vi "test_read-nmea-data2.vi"() -> ()   [LabVIEW 2019] (continued)
\tF9P\t\t\n15:11:49.05\tF9P\t\t\n15:11:49.07\tF9P\t\t\n15:11:49.09\tF9P\t\t\n15:11:49.11\tF9P\t\t\n15:11:49.13\tF9P\t\t\n15:11:49.15\tF9P\t\t\n15:11:49.17\tF9P\t\t\n15:11:49.19\tF9P\t\t\n15:11:49.21\tF9P\t\t\n15:11:49.23\tF9P\t\t\n15:11:49.25\tF9P\t$GNRMC,061151.00,A,3723.52582,N,12656.91812,E,3.101,50.80,250720,,,A,V*3C\n\t\n15:11:49.27\tF9P\t$GNVTG,50.80,T,,M,3.101,N,5.743,K,A*18\n\t\n15:11:49.29\tF9P\t$GNGGA,061151.00,3723.52582,N,12656.91812,E,1,12,0.68,36.2,M,18.5,M,,*7E\n\t\n15:11:49.31\tF9P\t$GNGSA,A,3,12,06,19,05,17,09,04,02,,,,,1.27,0.68,1.08,1*03\n\t\n15:11:49.33\tF9P\t$GNGSA,A,3,85,71,84,,,,,,,,,,1.27,0.68,1.08,2*06\n\t\n15:11:49.35\tF9P\t$GNGSA,A,3,36,19,11,04,09,12,,,,,,,1.27,0.68,1.08,3*03\n\t\n15:11:49.37\tF9P\t$GNGSA,A,3,14,11,33,,,,,,,,,,1.27,0.68,1.08,4*02\n\t\n15:11:49.39\tF9P\t$GPGSV,3,1,09,02,54,318,38,04,18,044,21,05,37,247,31,06,64,047,31,1*64\n\t\n15:11:49.41\tF9P\t$GPGSV,3,2,09,09,45,074,30,12,24,277,31,17,33,153,31,19,53,157,32,1*6E\n\t\n15:11:49.43\tF9P\t$GPGSV,3,3,09,25,12,307,16,1*5A\n\t\n15:11:49.45\tF9P\t$GPGSV,3,1,09,02,54,318,,04,18,044,13,05,37,247,16,06,64,047,28,6*64\n\t\n15:11:49.47\tF9P\t$GPGSV,3,2,09,09,45,074,30,12,24,277,21,17,33,153,23,19,53,157,,6*6A\n\t\n15:11:49.49\tF9P\t$GPGSV,3,3,09,25,12,307,,6*5A\n\t\n15:11:49.51\tF9P\t$GLGSV,2,1,08,69,12,031,,70,71,039,,71,52,205,44,72,04,209,,1*7A\n\t\n15:11:49.53\tF9P\t$GLGSV,2,2,08,77,01,326,,84,20,122,11,85,70,067,38,86,37,330,,1*73\n\t\n15:11:49.55\tF9P\t$GLGSV,2,1,08,69,12,031,,70,71,039,,71,52,205,21,72,04,209,,3*7B\n\t\n15:11:49.57\tF9P\t$GLGSV,2,2,08,77,01,326,,84,20,122,15,85,70,067,22,86,37,330,,3*7E\n\t\n15:11:49.59\tF9P\t$GAGSV,2,1,08,02,08,297,10,04,66,118,28,09,32,193,34,11,71,358,26,7*71\n\t\n15:11:49.61\tF9P\t$GAGSV,2,2,08,12,40,102,27,19,26,045,32,25,09,249,,36,26,308,32,7*7C\n\t\n15:11:49.63\tF9P\t$GAGSV,2,1,08,02,08,297,,04,66,118,,09,32,193,32,11,71,358,,2*7D\n\t\n15:11:49.65\tF9P\t$GAGSV,2,2,08,12,40,102,,19,26,045,,25,09,249,,36,26,308,,2*7C\n\t\n15:11:49.67\tF9P\t$GBGSV,1,1,03,11,50,132,31,14,87,127,28,33,60,219,34,1*4D\n\t\n15:11:49.69\tF9P\t$GBGSV,1,1,03,11,50,132,28,14,87,127,35,33,60,219,,3*4C\n\t\n15:11:49.71\tF9P\t$GNGLL,3723.52582,N,12656.91812,E,061151.00,A,A*7D\n\t\n15:11:49.73\tF9P\t\t\n15:11:49.75\tF9P\t\t\n15:11:49.77\tF9P\t\t\n15:11:49.79\tF9P\t\t\n15:11:49.81\tF9P\t\t\n15:11:49.83\tF9P\t\t\n15:11:49.85\tF9P\t\t\n15:11:49.87\tF9P\t\t\n15:11:49.89\tF9P\t\t\n15:11:49.91\tF9P\t\t\n15:11:49.93\tF9P\t\t\n15:11:49.95\tF9P\t\t\n15:11:49.97\tF9P\t\t\n15:11:49.99\tF9P\t\t\n15:11:50.01\tF9P\t\t\n15:11:50.03\tF9P\t\t\n15:11:50.05\tF9P\t\t\n15:11:50.07\tF9P\t\t\n15:11:50.09\tF9P\t\t\n15:11:50.11\tF9P\t\t\n15:11:50.13\tF9P\t\t\n15:11:50.15\tF9P\t\t\n15:11:50.17\tF9P\t\t\n15:11:50.19\tF9P\t\t\n15:11:50.21\tF9P\t\t\n15:11:50.23\tF9P\t\t\n15:11:50.25\tF9P\t$GNRMC,061152.00,A,3723.52625,N,12656.91894,E,2.824,51.00,250720,,,A,V*39\n\t\n15:11:50.27\tF9P\t$GNVTG,51.00,T,,M,2.824,N,5.229,K,A*17\n\t\n15:11:50.29\tF9P\t$GNGGA,061152.00,3723.52625,N,12656.91894,E,1,12,0.68,35.8,M,18.5,M,,*74\n\t\n15:11:50.31\tF9P\t$GNGSA,A,3,12,06,19,05,17,09,04,02,,,,,1.27,0.68,1.08,1*03\n\t\n15:11:50.33\tF9P\t$GNGSA,A,3,85,71,84,,,,,,,,,,1.27,0.68,1.08,2*06\n\t\n15:11:50.35\tF9P\t$GNGSA,A,3,36,19,11,04,09,12,,,,,,,1.27,0.68,1.08,3*03\n\t\n15:11:50.37\tF9P\t$GNGSA,A,3,14,11,33,,,,,,,,,,1.27,0.68,1.08,4*02\n\t\n15:11:50.39\tF9P\t$GPGSV,3,1,09,02,54,318,39,04,18,044,,05,37,247,26,06,64,047,32,1*63\n\t\n15:11:50.41\tF9P\t$GPGSV,3,2,09,09,45,074,30,12,24,277,28,17,33,153,30,19,53,157,34,1*61\n\t\n15:11:50.43\tF9P\t$GPGSV,3,3,09,25,12,307,17,1*5B\n\t\n15:11:50.45\tF9P\t$GPGSV,3,1,09,02,54,318,,04,18,044,14,05,37,247,17,06,64,047,29,6*63\n\t\n15:11:50.47\tF9P\t$GPGSV,3,2,09,09,45,074,32,12,24,277,20,17,33,153,24,19,53,157,,6*6E\n\t\n15:11:50.49\tF9P\t$GPGSV,3,3,09,25,12,307,,6*5A\n\t\n15:11:50.51\tF9P\t$GLGSV,2,1,08,69,12,031,,70,71,039,,71,52,205,48,72,04,209,,1*76\n\t\n15:11:50.53\tF9P\t$GLGSV,2,2,08,77,01,326,,84,20,122,12,85,70,067,35,86,37,330,,1*7D\n\t\n15:11:50.55\tF9P\t$GLGSV,2,1,08,69,12,031,,70,71,039,,71,52,205,22,72,04,209,,3*78\n\t\n15:11:50.57\tF9P\t$GLGSV,2,2,08,77,01,326,,84,20,122,15,85,70,067,21,86,37,330,,3*7D\n\t\n15:11:50.59\tF9P\t$GAGSV,2,1,08,02,08,297,08,04,66,118,29,09,32,193,34,11,71,358,26,7*79\n\t\n15:11:50.61\tF9P\t$GAGSV,2,2,08,12,40,102,26,19,26,045,31,25,09,249,,36,26,308,23,7*7E\n\t\n15:11:50.63\tF9P\t$GAGSV,2,1,08,02,08,297,,04,66,118,,09,32,193,33,11,71,358,,2*7C\n\t\n15:11:50.65\tF9P\t$GAGSV,2,2,08,12,40,102,,19,26,045,,25,09,249,,36,26,308,,2*7C\n\t\n15:11:50.67\tF9P\t$GBGSV,1,1,03,11,50,132,30,14,87,127,32,33,60,219,37,1*44\n\t\n15:11:50.69\tF9P\t$GBGSV,1,1,03,11,50,132,,14,87,127,,33,60,219,,3*40\n\t\n15:11:50.71\tF9P\t$GNGLL,3723.52625,N,12656.91894,E,061152.00,A,A*7E\n\t\n15:11:50.73\tF9P\t\t\n15:11:50.75\tF9P\t\t\n15:11:50.77\tF9P\t\t\n15:11:50.79\tF9P\t\t\n15:11:50.81\tF9P\t\t\n15:11:50.83\tF9P\t\t\n15:11:50.85\tF9P\t\t\n15:11:50.87\tF9P\t\t\n15:11:50.89\tF9P\t\t\n15:11:50.91\tF9P\t\t\n15:11:50.93\tF9P\t\t\n15:11:50.95\tF9P\t\t\n15:11:50.97\tF9P\t\t\n15:11:50.99\tF9P\t\t\n15:11:51.01\tF9P\t\t\n15:11:51.03\tF9P\t\t\n15:11:51.05\tF9P\t\t\n15:11:51.07\tF9P\t\t\n15:11:51.09\tF9P\t\t\n15:11:51.11\tF9P\t\t\n15:11:51.13\tF9P\t\t\n15:11:51.15\tF9P\t\t\n15:11:51.17\tF9P\t\t\n15:11:51.19\tF9P\t\t\n15:11:51.21\tF9P\t\t\n15:11:51.23\tF9P\t\t\n15:11:51.25\tF9P\t$GNRMC,061153.00,A,3723.52665,N,12656.91962,E,2.290,47.20,250720,,,A,V*34\n\t\n15:11:51.27\tF9P\t$GNVTG,47.20,T,,M,2.290,N,4.241,K,A*18\n\t\n15:11:51.29\tF9P\t$GNGGA,061153.00,3723.52665,N,12656.91962,E,1,12,0.71,35.0,M,18.5,M,,*79\n\t\n15:11:51.31\tF9P\t$GNGSA,A,3,12,06,19,05,17,09,04,02,,,,,1.31,0.71,1.10,1*05\n\t\n15:11:51.33\tF9P\t$GNGSA,A,3,85,71,84,,,,,,,,,,1.31,0.71,1.10,2*00\n\t\n15:11:51.35\tF9P\t$GNGSA,A,3,36,19,11,04,09,12,,,,,,,1.31,0.71,1.10,3*05\n\t\n15:11:51.37\tF9P\t$GNGSA,A,3,14,11,33,,,,,,,,,,1.31,0.71,1.10,4*04\n\t\n15:11:51.39\tF9P\t$GPGSV,3,1,09,02,54,318,41,04,18,044,23,05,37,247,26,06,64,047,32,1*6D\n\t\n15:11:51.41\tF9P\t$GPGSV,3,2,09,09,45,074,34,12,24,277,28,17,33,153,34,19,53,157,33,1*66\n\t\n15:11:51.43\tF9P\t$GPGSV,3,3,09,25,12,307,16,1*5A\n\t\n15:11:51.45\tF9P\t$GPGSV,3,1,09,02,54,318,,04,18,044,15,05,37,247,16,06,64,047,32,6*69\n\t\n15:11:51.47\tF9P\t$GPGSV,3,2,09,09,45,074,26,12,24,277,18,17,33,153,23,19,53,157,,6*67\n\t\n15:11:51.49\tF9P\t$GPGSV,3,3,09,25,12,307,,6*5A\n\t\n15:11:51.51\tF9P\t$GLGSV,2,1,08,69,12,031,,70,71,039,,71,52,205,41,72,04,209,,1*7F\n\t\n15:11:51.53\tF9P\t$GLGSV,2,2,08,77,01,326,,84,20,122,11,85,70,067,31,86,37,330,,1*7A\n\t\n15:11:51.55\tF9P\t$GLGSV,2,1,08,69,12,031,,70,71,039,,71,52,205,24,72,04,209,,3*7E\n\t\n15:11:51.57\tF9P\t$GLGSV,2,2,08,77,01,326,,84,20,122,15,85,70,067,29,86,37,330,,3*75\n\t\n15:11:51.59\tF9P\t$GAGSV,2,1,08,02,08,297,12,04,66,118,29,09,32,193,37,11,71,358,31,7*77\n\t\n15:11:51.61\tF9P\t$GAGSV,2,2,08,12,40,102,32,19,26,045,24,25,09,249,,36,26,308,30,7*7D\n\t\n15:11:51.63\tF9P\t$GAGSV,2,1,08,02,08,297,,04,66,118,,09,32,193,,11,71,358,,2*7C\n\t\n15:11:51.65\tF9P\t$GAGSV,2,2,08,12,40,102,,19,26,045,,25,09,249,,36,26,308,,2*7C\n\t\n15:11:51.67\tF9P\t$GBGSV,1,1,03,11,50,132,24,14,87,127,33,33,60,219,38,1*4F\n\t\n15:11:51.69\tF9P\t$GBGSV,1,1,04,08,,,32,11,50,132,,14,87,127,,33,60,219,,3*4E\n\t\n15:11:51.71\tF9P\t$GNGLL,3723.52665,N,12656.91962,E,061153.00,A,A*73\n\t\n15:11:51.73\tF9P\t\t\n15:11:51.75\tF9P\t\t\n15:11:51.77\tF9P\t\t\n15:11:51.79\tF9P\t\t\n15:11:51.81\tF9P\t\t\n15:11:51.83\tF9P\t\t\n15:11:51.85\tF9P\t\t\n15:11:51.87\tF9P\t\t\n15:11:51.89\tF9P\t\t\n15:11:51.91\tF9P\t\t\n15:11:51.93\tF9P\t\t\n15:11:51.95\tF9P\t\t\n15:11:51.97\tF9P\t\t\n15:11:51.99\tF9P\t\t\n15:11:52.01\tF9P\t\t\n15:11:52.03\tF9P\t\t\n15:11:52.05\tF9P\t\t\n15:11:52.07\tF9P\t\t\n15:11:52.09\tF9P\t\t\n15:11:52.11\tF9P\t\t\n15:11:52.13\tF9P\t\t\n15:11:52.15\tF9P\t\t\n15:11:52.17\tF9P\t\t\n15:11:52.19\tF9P\t\t\n15:11:52.21\tF9P\t\t\n15:11:52.23\tF9P\t\t\n15:11:52.25\tF9P\t$GNRMC,061154.00,A,3723.52702,N,12656.92007,E,2.069,41.23,250720,,,A,V*3B\n\t\n15:11:52.27\tF9P\t$GNVTG,41.23,T,,M,2.069,N,3.832,K,A*10\n\t\n15:11:52.29\tF9P\t$GNGGA,061154.00,3723.52702,N,12656.92007,E,1,12,0.68,35.3,M,18.5,M,,*7C\n\t\n15:11:52.31\tF9P\t$GNGSA,A,3,12,06,19,05,17,09,04,02,,,,,1.27,0.68,1.08,1*03\n\t\n15:11:52.33\tF9P\t$GNGSA,A,3,85,71,84,,,,,,,,,,1.27,0.68,1.08,2*06\n\t\n15:11:52.35\tF9P\t$GNGSA,A,3,36,19,11,04,09,12,,,,,,,1.27,0.68,1.08,3*03\n\t\n15:11:52.37\tF9P\t$GNGSA,A,3,14,11,33,,,,,,,,,,1.27,0.68,1.08,4*02\n\t\n15:11:52.39\tF9P\t$GPGSV,3,1,09,02,55,319,43,04,18,044,22,05,37,247,27,06,64,047,33,1*6E\n\t\n15:11:52.41\tF9P\t$GPGSV,3,2,09,09,45,074,33,12,24,277,27,17,33,153,36,19,53,157,36,1*69\n\t\n15:11:52.43\tF9P\t$GPGSV,3,3,09,25,12,307,18,1*54\n\t\n15:11:52.45\tF9P\t$GPGSV,3,1,09,02,55,319,,04,18,044,17,05,37,247,15,06,64,047,27,6*6C\n\t\n15:11:52.47\tF9P\t$GPGSV,3,2,09,09,45,074,28,12,24,277,17,17,33,153,23,19,53,157,,6*66\n\t\n15:11:52.49\tF9P\t$GPGSV,3,3,09,25,12,307,,6*5A\n\t\n15:11:52.51\tF9P\t$GLGSV,2,1,08,69,12,031,,70,71,039,,71,52,205,44,72,04,209,,1*7A\n\t\n15:11:52.53\tF9P\t$GLGSV,2,2,08,77,01,326,,84,20,122,12,85,70,067,35,86,37,330,,1*7D\n\t\n15:11:52.55\tF9P\t$GLGSV,2,1,08,69,12,031,,70,71,039,,71,52,205,30,72,04,209,,3*7B\n\t\n15:11:52.57\tF9P\t$GLGSV,2,2,08,77,01,326,,84,20,122,15,85,70,067,28,86,37,330,,3*74\n\t\n15:11:52.59\tF9P\t$GAGSV,2,1,08,02,08,297,08,04,66,118,28,09,32,193,43,11,71,358,26,7*78\n\t\n15:11:52.61\tF9P\t$GAGSV,2,2,08,12,40,102,26,19,26,045,24,25,09,249,,36,26,308,29,7*70\n\t\n15:11:52.63\tF9P\t$GAGSV,2,1,08,02,08,297,,04,66,118,,09,32,193,,11,71,358,,2*7C\n\t\n15:11:52.65\tF9P\t$GAGSV,2,2,08,12,40,102,,19,26,045,,25,09,249,,36,26,308,,2*7C\n\t\n15:11:52.67\tF9P\t$GBGSV,1,1,03,11,50,132,29,14,87,127,31,33,60,219,40,1*4F\n\t\n15:11:52.69\tF9P\t$GBGSV,1,1,04,08,,,27,11,50,132,,14,87,127,,33,60,219,,3*4A\n\t\n15:11:52.71\tF9P\t$GNGLL,3723.52702,N,12656.92007,E,061154.00,A,A*7D\n\t\n15:11:52.73\tF9P\t\t\n15:11:52.75\tF9P\t\t\n15:11:52.77\tF9P\t\t\n15:11:52.79\tF9P\t\t\n15:11:52.81\tF9P\t\t\n15:11:52.83\tF9P\t\t\n15:11:52.85\tF9P\t\t\n15:11:52.87\tF9P\t\t\n15:11:52.89\tF9P\t\t\n15:11:52.91\tF9P\t\t\n15:11:52.93\tF9P\t\t\n15:11:52.95\tF9P\t\t\n15:11:52.97\tF9P\t\t\n15:11:52.99\tF9P\t\t\n15:11:53.01\tF9P\t\t\n15:11:53.03\tF9P\t\t\n15:11:53.05\tF9P\t\t\n15:11:53.07\tF9P\t\t\n15:11:53.09\tF9P\t\t\n15:11:53.11\tF9P\t\t\n15:11:53.13\tF9P\t\t\n15:11:53.15\tF9P\t\t\n15:11:53.17\tF9P\t\t\n15:11:53.19\tF9P\t\t\n15:11:53.21\tF9P\t\t\n15:11:53.23\tF9P\t\t\n15:11:53.25\tF9P\t$GNRMC,061155.00,A,3723.52737,N,12656.92072,E,2.566,49.21,250720,,,A,V*3E\n\t\n15:11:53.27\tF9P\t$GNVTG,49.21,T,,M,2.566,N,4.751,K,A*1D\n\t\n15:11:53.29\tF9P\t$GNGGA,061155.00,3723.52737,N,12656.92072,E,1,12,0.70,34.5,M,18.5,M,,*77\n\t\n15:11:53.31\tF9P\t$GNGSA,A,3,12,06,19,05,17,09,04,02,,,,,1.39,0.70,1.20,1*0F\n\t\n15:11:53.33\tF9P\t$GNGSA,A,3,85,70,71,84,,,,,,,,,1.39,0.70,1.20,2*0D\n\t\n15:11:53.35\tF9P\t$GNGSA,A,3,36,19,11,04,09,12,,,,,,,1.39,0.70,1.20,3*0F\n\t\n15:11:53.37\tF9P\t$GNGSA,A,3,14,11,33,,,,,,,,,,1.39,0.70,1.20,4*0E\n\t\n15:11:53.39\tF9P\t$GPGSV,3,1,09,02,55,319,39,04,18,044,25,05,37,247,26,06,64,047,34,1*62\n\t\n15:11:53.41\tF9P\t$GPGSV,3,2,09,09,45,074,33,12,24,277,26,17,33,153,40,19,53,157,33,1*6C\n\t\n15:11:53.43\tF9P\t$GPGSV,3,3,09,25,12,307,17,1*5B\n\t\n15:11:53.45\tF9P\t$GPGSV,3,1,09,02,55,319,,04,18,044,15,05,37,247,14,06,64,047,26,6*6E\n\t\n15:11:53.47\tF9P\t$GPGSV,3,2,09,09,45,074,33,12,24,277,14,17,33,153,24,19,53,157,,6*68\n\t\n15:11:53.49\tF9P\t$GPGSV,3,3,09,25,12,307,,6*5A\n\t\n15:11:53.51\tF9P\t$GLGSV,2,1,08,69,12,031,,70,71,039,32,71,52,205,45,72,04,209,,1*7A\n\t\n15:11:53.53\tF9P\t$GLGSV,2,2,08,77,01,326,,84,20,122,11,85,70,067,29,86,37,330,,1*73\n\t\n15:11:53.55\tF9P\t$GLGSV,2,1,08,69,12,031,,70,71,039,,71,52,205,30,72,04,209,,3*7B\n\t\n15:11:53.57\tF9P\t$GLGSV,2,2,08,77,01,326,,84,20,122,17,85,70,067,26,86,37,330,,3*78\n\t\n15:11:53.59\tF9P\t$GAGSV,2,1,08,02,08,297,12,04,66,118,29,09,32,193,33,11,71,358,26,7*75\n\t\n15:11:53.61\tF9P\t$GAGSV,2,2,08,12,40,102,27,19,26,045,25,25,09,249,,36,26,308,33,7*7B\n\t\n15:11:53.63\tF9P\t$GAGSV,2,1,08,02,08,297,,04,66,118,,09,32,193,,11,71,358,,2*7C\n\t\n15:11:53.65\tF9P\t$GAGSV,2,2,08,12,40,102,,19,26,045,,25,09,249,,36,26,308,,2*7C\n\t\n15:11:53.67\tF9P\t$GBGSV,1,1,03,11,50,132,29,14,87,127,26,33,60,219,33,1*4D\n\t\n15:11:53.69\tF9P\t$GBGSV,1,1,04,08,,,25,11,50,132,,14,87,127,,33,60,219,,3*48\n\t\n15:11:53.71\tF9P\t$GNGLL,3723.52737,N,12656.92072,E,061155.00,A,A*78\n\t\n15:11:53.73\tF9P\t\t\n15:11:53.75\tF9P\t\t\n15:11:53.77\tF9P\t\t\n15:11:53.79\tF9P\t\t\n15:11:53.81\tF9P\t\t\n15:11:53.83\tF9P\t\t\n15:11:53.85\tF9P\t\t\n15:11:53.87\tF9P\t\t\n15:11:53.89\tF9P\t\t\n15:11:53.91\tF9P\t\t\n15:11:53.93\tF9P\t\t\n15:11:53.95\tF9P\t\t\n15:11:53.97\tF9P\t\t\n15:11:53.99\tF9P\t\t\n15:11:54.01\tF9P\t\t\n15:11:54.03\tF9P\t\t\n15:11:54.05\tF9P\t\t\n15:11:54.07\tF9P\t\t\n15:11:54.09\tF9P\t\t\n15:11:54.11\tF9P\t\t\n15:11:54.13\tF9P\t\t\n15:11:54.15\tF9P\t\t\n15:11:54.17\tF9P\t\t\n15:11:54.19\tF9P\t\t\n15:11:54.21\tF9P\t\t\n15:11:54.23\tF9P\t\t\n15:11:54.25\tF9P\t$GNRMC,061156.00,A,3723.52762,N,12656.92145,E,2.113,57.27,250720,,,A,V*37\n\t\n15:11:54.27\tF9P\t$GNVTG,57.27,T,,M,2.113,N,3.912,K,A*1C\n\t\n15:11:54.29\tF9P\t$GNGGA,061156.00,3723.52762,N,12656.92145,E,1,12,0.67,33.0,M,18.5,M,,*75\n\t\n15:11:54.31\tF9P\t$GNGSA,A,3,12,06,19,05,17,09,04,02,,,,,1.25,0.67,1.05,1*03\n\t\n15:11:54.33\tF9P\t$GNGSA,A,3,85,70,71,84,,,,,,,,,1.25,0.67,1.05,2*01\n\t\n15:11:54.35\tF9P\t$GNGSA,A,3,36,19,11,04,09,12,,,,,,,1.25,0.67,1.05,3*03\n\t\n15:11:54.37\tF9P\t$GNGSA,A,3,14,11,33,,,,,,,,,,1.25,0.67,1.05,4*02\n\t\n15:11:54.39\tF9P\t$GPGSV,3,1,09,02,55,319,33,04,18,043,22,05,37,247,25,06,64,047,36,1*69\n\t\n15:11:54.41\tF9P\t$GPGSV,3,2,09,09,45,074,41,12,24,277,26,17,33,153,41,19,53,157,30,1*6B\n\t\n15:11:54.43\tF9P\t$GPGSV,3,3,09,25,12,307,17,1*5B\n\t\n15:11:54.45\tF9P\t$GPGSV,3,1,09,02,55,319,,04,18,043,15,05,37,247,15,06,64,047,31,6*6E\n\t\n15:11:54.47\tF9P\t$GPGSV,3,2,09,09,45,074,34,12,24,277,14,17,33,153,24,19,53,157,,6*6F\n\t\n15:11:54.49\tF9P\t$GPGSV,3,3,09,25,12,307,,6*5A\n\t\n15:11:54.51\tF9P\t$GLGSV,2,1,08,69,12,031,,70,71,039,33,71,52,205,39,72,04,209,,1*70\n\t\n15:11:54.53\tF9P\t$GLGSV,2,2,08,77,01,326,,84,20,122,11,85,70,067,36,86,37,330,,1*7D\n\t\n15:11:54.55\tF9P\t$GLGSV,2,1,08,69,12,031,,70,71,039,,71,52,205,30,72,04,209,,3*7B\n\t\n15:11:54.57\tF9P\t$GLGSV,2,2,08,77,01,326,,84,20,122,19,85,70,067,26,86,37,330,,3*76\n\t\n15:11:54.59\tF9P\t$GAGSV,2,1,08,02,08,297,07,04,66,118,30,09,32,193,33,11,71,358,31,7*7F\n\t\n15:11:54.61\tF9P\t$GAGSV,2,2,08,12,40,102,28,19,26,045,25,25,09,249,,36,26,308,33,7*74\n\t\n15:11:54.63\tF9P\t$GAGSV,2,1,08,02,08,297,,04,66,118,,09,32,193,,11,71,358,,2*7C\n\t\n15:11:54.65\tF9P\t$GAGSV,2,2,08,12,40,102,,19,26,045,,25,09,249,,36,26,308,,2*7C\n\t\n15:11:54.67\tF9P\t$GBGSV,1,1,03,11,50,132,29,14,87,127,35,33,60,219,40,1*4B\n\t\n15:11:54.69\tF9P\t$GBGSV,1,1,03,11,50,132,27,14,87,127,,33,60,219,,3*45\n\t\n15:11:54.71\tF9P\t$GNGLL,3723.52762,N,12656.92145,E,061156.00,A,A*7E\n\t\n15:11:54.73\tF9P\t\t\n15:11:54.75\tF9P\t\t\n15:11:54.77\tF9P\t\t\n15:11:54.79\tF9P\t\t\n15:11:54.81\tF9P\t\t\n15:11:54.83\tF9P\t\t\n15:11:54.85\tF9P\t\t\n15:11:54.87\tF9P\t\t\n15:11:54.89\tF9P\t\t\n15:11:54.91\tF9P\t\t\n15:11:54.93\tF9P\t\t\n15:11:54.95\tF9P\t\t\n15:11:54.97\tF9P\t\t\n15:11:54.99\tF9P\t\t\n15:11:55.01\tF9P\t\t\n15:11:55.03\tF9P\t\t\n15:11:55.05\tF9P\t\t\n15:11:55.07\tF9P\t\t\n15:11:55.09\tF9P\t\t\n15:11:55.11\tF9P\t\t\n15:11:55.13\tF9P\t\t\n15:11:55.15\tF9P\t\t\n15:11:55.17\tF9P\t\t\n15:11:55.19\tF9P\t\t\n15:11:55.21\tF9P\t\t\n15:11:55.23\tF9P\t\t\n15:11:55.25\tF9P\t$GNRMC,061157.00,A,3723.52794,N,12656.92203,E,2.654,43.75,250720,,,A,V*38\n\t\n15:11:55.27\tF9P\t$GNVTG,43.75,T,,M,2.654,N,4.915,K,A*1A\n\t\n15:11:55.29\tF9P\t$GNGGA,061157.00,3723.52794,N,12656.92203,E,1,12,0.67,33.5,M,18.5,M,,*79\n\t\n15:11:55.31\tF9P\t$GNGSA,A,3,12,06,19,05,17,09,04,02,,,,,1.25,0.67,1.05,1*03\n\t\n15:11:55.33\tF9P\t$GNGSA,A,3,85,70,71,84,,,,,,,,,1.25,0.67,1.05,2*01\n\t\n15:11:55.35\tF9P\t$GNGSA,A,3,36,19,11,04,09,12,,,,,,,1.25,0.67,1.05,3*03\n\t\n15:11:55.37\tF9P\t$GNGSA,A,3,14,11,33,,,,,,,,,,1.25,0.67,1.05,4*02\n\t\n15:11:55.39\tF9P\t$GPGSV,3,1,09,02,55,319,39,04,18,043,21,05,37,247,25,06,64,047,36,1*60\n\t\n15:11:55.41\tF9P\t$GPGSV,3,2,09,09,45,074,39,12,24,277,26,17,33,153,34,19,53,157,31,1*67\n\t\n15:11:55.43\tF9P\t$GPGSV,3,3,09,25,12,307,16,1*5A\n\t\n15:11:55.45\tF9P\t$GPGSV,3,1,09,02,55,319,,04,18,043,16,05,37,247,16,06,64,047,25,6*6B\n\t\n15:11:55.47\tF9P\t$GPGSV,3,2,09,09,45,074,34,12,24,277,13,17,33,153,23,19,53,157,,6*6F\n\t\n15:11:55.49\tF9P\t$GPGSV,3,3,09,25,12,307,,6*5A\n\t\n15:11:55.51\tF9P\t$GLGSV,2,1,08,69,12,031,,70,71,039,36,71,52,205,42,72,04,209,,1*79\n\t\n15:11:55.53\tF9P\t$GLGSV,2,2,08,77,01,326,,84,20,122,12,85,70,067,40,86,37,330,,1*7F\n\t\n15:11:55.55\tF9P\t$GLGSV,2,1,08,69,12,031,,70,71,039,,71,52,205,29,72,04,209,,3*73\n\t\n15:11:55.57\tF9P\t$GLGSV,2,2,08,77,01,326,,84,20,122,18,85,70,067,26,86,37,330,,3*77\n\t\n15:11:55.59\tF9P\t$GAGSV,2,1,08,02,08,297,09,04,66,118,29,09,32,193,41,11,71,358,25,7*79\n\t\n15:11:55.61\tF9P\t$GAGSV,2,2,08,12,40,102,28,19,26,045,25,25,09,249,,36,26,308,28,7*7E\n\t\n15:11:55.63\tF9P\t$GAGSV,2,1,08,02,08,297,,04,66,118,,09,32,193,,11,71,358,,2*7C\n\t\n15:11:55.65\tF9P\t$GAGSV,2,2,08,12,40,102,,19,26,045,,25,09,249,,36,26,308,,2*7C\n\t\n15:11:55.67\tF9P\t$GBGSV,1,1,03,11,50,132,29,14,87,127,28,33,60,219,39,1*49\n\t\n15:11:55.69\tF9P\t$GBGSV,1,1,03,11,50,132,,14,87,127,,33,60,219,,3*40\n\t\n15:11:55.71\tF9P\t$GNGLL,3723.52794,N,12656.92203,E,061157.00,A,A*77\n\t\n15:11:55.73\tF9P\t\t\n15:11:55.75\tF9P\t\t\n15:11:55.77\tF9P\t\t\n15:11:55.79\tF9P\t\t\n15:11:55.81\tF9P\t\t\n15:11:55.83\tF9P\t\t\n15:11:55.85\tF9P\t\t\n15:11:55.87\tF9P\t\t\n15:11:55.89\tF9P\t\t\n15:11:55.91\tF9P\t\t\n15:11:55.93\tF9P\t\t\n15:11:55.95\tF9P\t\t\n15:11:55.97\tF9P\t\t\n15:11:55.99\tF9P\t\t\n15:11:56.01\tF9P\t\t\n15:11:56.03\tF9P\t\t\n15:11:56.05\tF9P\t\t\n15:11:56.07\tF9P\t\t\n15:11:56.09\tF9P\t\t\n15:11:56.11\tF9P\t\t\n15:11:56.13\tF9P\t\t\n15:11:56.15\tF9P\t\t\n15:11:56.17\tF9P\t\t\n15:11:56.19\tF9P\t\t\n15:11:56.21\tF9P\t\t\n15:11:56.23\tF9P\t\t\n15:11:56.25\tF9P\t$GNRMC,061158.00,A,3723.52845,N,12656.92271,E,2.934,44.91,250720,,,A,V*35\n\t\n15:11:56.27\tF9P\t$GNVTG,44.91,T,,M,2.934,N,5.434,K,A*11\n\t\n15:11:56.29\tF9P\t$GNGGA,061158.00,3723.52845,N,12656.92271,E,1,12,0.70,33.4,M,18.5,M,,*77\n\t\n15:11:56.31\tF9P\t$GNGSA,A,3,12,06,19,05,17,09,04,02,,,,,1.39,0.70,1.20,1*0F\n\t\n15:11:56.33\tF9P\t$GNGSA,A,3,85,70,71,84,,,,,,,,,1.39,0.70,1.20,2*0D\n\t\n15:11:56.35\tF9P\t$GNGSA,A,3,36,19,11,04,09,12,,,,,,,1.39,0.70,1.20,3*0F\n\t\n15:11:56.37\tF9P\t$GNGSA,A,3,14,11,33,,,,,,,,,,1.39,0.70,1.20,4*0E\n\t\n15:11:56.39\tF9P\t$GPGSV,3,1,09,02,55,319,41,04,18,043,,05,37,247,25,06,64,049,31,1*65\n\t\n15:11:56.41\tF9P\t$GPGSV,3,2,09,09,45,074,35,12,24,277,25,17,33,153,37,19,53,157,33,1*69\n\t\n15:11:56.43\tF9P\t$GPGSV,3,3,09,25,12,307,16,1*5A\n\t\n15:11:56.45\tF9P\t$GPGSV,3,1,09,02,55,319,,04,18,043,16,05,37,247,15,06,64,049,26,6*65\n\t\n15:11:56.47\tF9P\t$GPGSV,3,2,09,09,45,074,26,12,24,277,13,17,33,153,25,19,53,157,,6*6A\n\t\n15:11:56.49\tF9P\t$GPGSV,3,3,09,25,12,307,,6*5A\n\t\n15:11:56.51\tF9P\t$GLGSV,2,1,08,69,12,031,,70,71,039,28,71,52,205,37,72,04,209,,1*74\n\t\n15:11:56.53\tF9P\t$GLGSV,2,2,08,77,01,326,,84,20,122,13,85,70,067,33,86,37,330,,1*7A\n\t\n15:11:56.55\tF9P\t$GLGSV,2,1,08,69,12,031,,70,71,039,,71,52,205,29,72,04,209,,3*73\n\t\n15:11:56.57\tF9P\t$GLGSV,2,2,08,77,01,326,,84,20,122,18,85,70,067,24,86,37,330,,3*75\n\t\n15:11:56.59\tF9P\t$GAGSV,2,1,08,02,08,297,08,04,66,118,29,09,32,193,35,11,71,358,26,7*78\n\t\n15:11:56.61\tF9P\t$GAGSV,2,2,08,12,40,102,28,19,26,045,25,25,09,249,,36,26,308,20,7*76\n\t\n15:11:56.63\tF9P\t$GAGSV,2,1,08,02,08,297,,04,66,118,,09,32,193,,11,71,358,,2*7C\n\t\n15:11:56.65\tF9P\t$GAGSV,2,2,08,12,40,102,,19,26,045,,25,09,249,,36,26,308,,2*7C\n\t\n15:11:56.67\tF9P\t$GBGSV,1,1,03,11,50,132,29,14,87,127,29,33,60,219,32,1*43\n\t\n15:11:56.69\t
